vi "get cell width.vi"(7 "T: Barcode Length\nF: Barcode string":bool, 10 "Barcode length":i32, 11 "String Input":string) -> (3 "Cell Size:Width":u32)   [LabVIEW 2021]
doc: "在默认15字体的情况下，根据输入的字符串长度绝对单元格的宽度。\n# 2020-7-13 09:40:13"
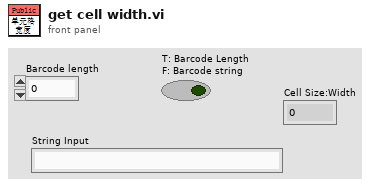
[diagram p1: front panel]
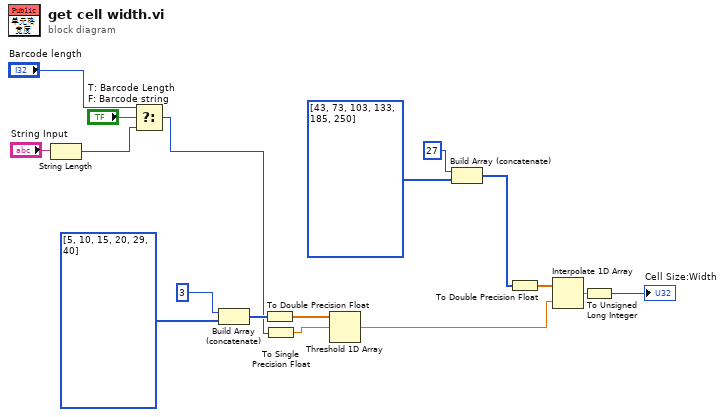
[diagram p0: block diagram]
diagram:
  n1 = String Length(string="String Input") -> (length=w4:i32)
  n2 = Select(t="Barcode length", s="T: Barcode Length\nF: Barcode string", f=w4) -> (s? t:f=w3:i32)
  n3 = Build Array (concatenate)(3, i32[] [5, 10, 15, 20, 29, 40]) -> (w14:i32[])
  n4 = To Double Precision Float(number=w14) -> (double precision float=w8:dbl[])
  n5 = To Single Precision Float(number=w3) -> (single precision float=w9:sgl)
  n6 = Threshold 1D Array(2:w9, 3:w8) -> (0:w12:dbl)  [unwired: 1 in]
  n7 = Build Array (concatenate)(27, i32[] [43, 73, 103, 133, 185, 250]) -> (w16:i32[])
  n8 = To Double Precision Float(number=w16) -> (double precision float=w11:dbl[])
  n9 = Interpolate 1D Array(1:w12, 2:w11) -> (0:w13:dbl)
  n10 = To Unsigned Long Integer(number=w13) -> (unsigned 32bit integer=→"Cell Size:Width":u32)
